vi "串口配置.vi"(10 "波特率":u32(ring)=115200 caption="波特率：" items=["9600"=9600, "19200"=19200, "115200"=115200], 11 "VISA资源名称":refnum<visa-resource-name>) -> (1 "确认 2":bool, 2 "波特率 2":u32(ring)=115200 caption="波特率：" items=["9600"=9600, "19200"=19200, "115200"=115200], 3 "VISA资源名称 2":refnum<visa-resource-name>)   [LabVIEW 2016, in "斯坦道多参数.lvlib"]
panel:
  in  "取消":bool
  in  "确认":bool
  # "请选择串口:"
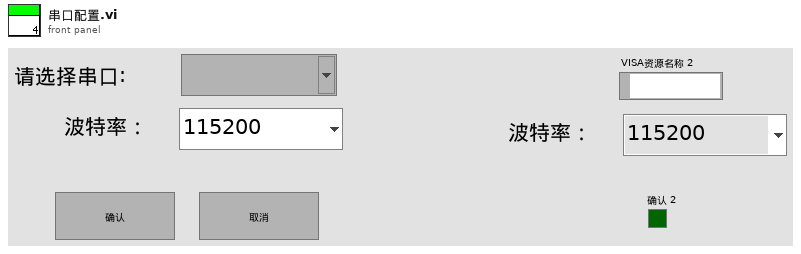
[diagram p1: front panel]
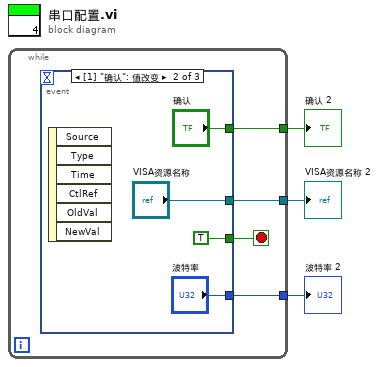
[diagram p0: block diagram]
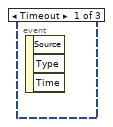
[diagram p2: hidden frame]
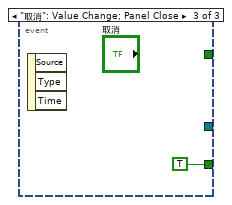
[diagram p3: hidden frame]
diagram:
  n1 = while {
    tunnel: [w7] -> w3
    tunnel: [w5] -> w2
    tunnel: [w4] -> w1
    stop <- w6 stop-if-true
    n2 = event shown="[1] \"确认\": 值改变" {
      selector: _ -> [_ _ _]
      dyn-events: _ -> [_ _ _]
      timeout: _ -> [_ _ _]
      tunnel: [_ "VISA资源名称" _] -> w7
      tunnel: [_ TRUE TRUE] -> w6
      tunnel: [_ "确认" _] -> w5
      tunnel: [_ "波特率" _] -> w4
      event Timeout {
        n3 = event-data() -> ()  [unwired: 1 in, 3 out]
      }
      event "确认": Value Change {
        n4 = event-data() -> ()  [unwired: 1 in, 6 out]
      }
      event "取消": Value Change; Panel Close {
        n5 = event-data() -> ()  [unwired: 1 in, 3 out]
      }
    }
  }
  "VISA资源名称 2" <- w3
  "确认 2" <- w2
  "波特率 2" <- w1
